vi "Set File Type.vi"(10 "Value":T2, 11 "App Data In":T1) -> (3 "App Data Out":T1)   [LabVIEW 2019]
uses:
  TypeDef/File Type.ctl
  TypeDef/App Data.ctl
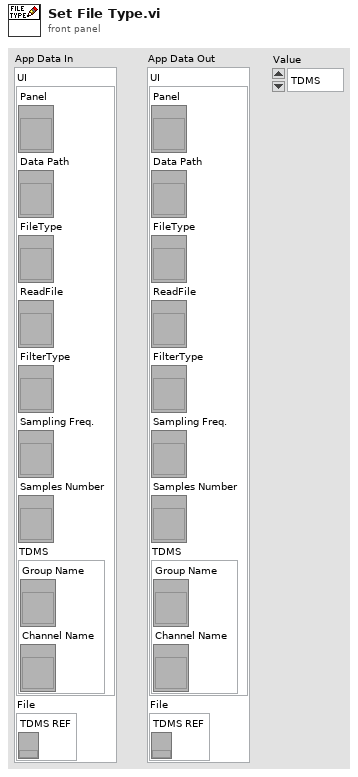
[diagram p1: front panel]
types:
  T1 = typedef "App Data.ctl" = cluster{"UI":cluster{"Panel":refnum<vi>, "Data Path":refnum<vi>, "FileType":refnum<vi>, "ReadFile":refnum<vi>, "FilterType":refnum<vi>, "Sampling Freq.":refnum<vi>, "Samples Number":refnum<vi>, "TDMS":cluster{"Group Name":refnum<vi>, "Channel Name":refnum<vi>}}, "File":cluster{"TDMS REF":refnum<k34>}}
  T2 = typedef "File Type.ctl" = enum32{"TDMS", "CSV"}
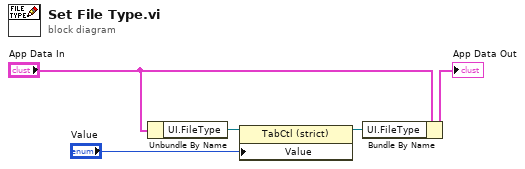
[diagram p0: block diagram]
diagram:
  n1 = Unbundle By Name("App Data In") -> ("UI.FileType"=w3:refnum<vi>)
  n2 = property class="TabCtl (strict)"(reference=w3, "Value"="Value") -> (reference out=w4:refnum<vi>)  [unwired: 1 in, 1 out]
  n3 = Bundle By Name(cluster="App Data In", "UI.FileType"=w4) -> (→"App Data Out":T1)
